vi "Set_Deploy_EXE_Data.vi"(8 "error in (no error)":errorcluster, 10 "data":T1, 11 "AB_Deploy_EXE.lvclass in":refnum<class "AB_Deploy_EXE.lvclass">) -> (0 "error out":errorcluster, 3 "AB_Deploy_EXE.lvclass out":refnum<class "AB_Deploy_EXE.lvclass">)   [LabVIEW 2020, in "AB_Deploy_EXE.lvclass"]
uses:
  <vilib>/AppBuilder/AB_Classes/DeployableEXE/AB_Deploy_EXE.lvclass
  <vilib>/AppBuilder/AB_Classes/DeployableEXE/AB_Deploy_EXE.lvclass/AB_Deploy_EXE.ctl
  <vilib>/AppBuilder/AB_Classes/DeployableEXE/AB_Deploy_EXE.ctl
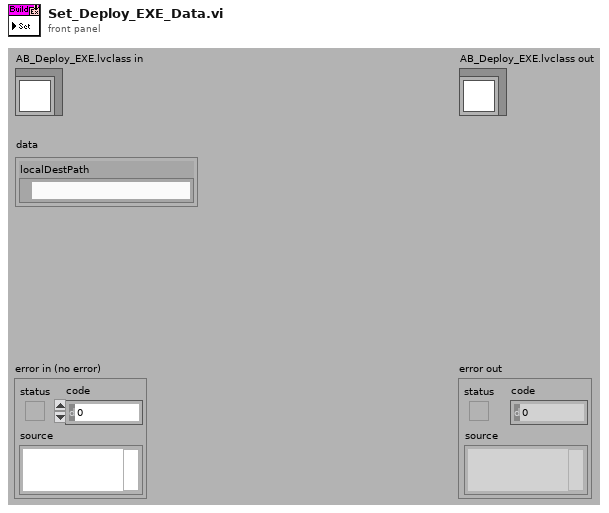
[diagram p1: front panel]
types:
  T1 = typedef "AB_Deploy_EXE.ctl" = cluster{"localDestPath":path}
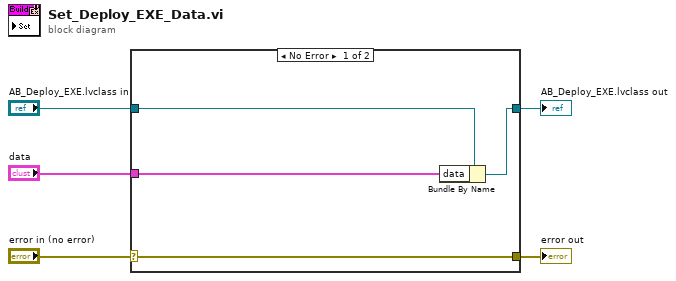
[diagram p0: block diagram]
diagram:
  n1 = case shown="No Error" "error in (no error)" {
    selector: "error in (no error)" -> [w9 w10]
    tunnel: [w9 w10] -> w4
    tunnel: [w7 w11] -> w2
    tunnel: "AB_Deploy_EXE.lvclass in" -> [w8 w11]
    tunnel: "data" -> [w6 _]
    frame No Error {
      n2 = Bundle By Name(cluster=w8, "data"=w6) -> (w7:refnum<class "AB_Deploy_EXE.lvclass">)
    }
    frame Error {
    }
  }
  "error out" <- w4
  "AB_Deploy_EXE.lvclass out" <- w2
